vi "write includes file path.vi"(8 "error in":errorcluster, 10 "Path":path, 11 "Targets in":refnum<class "Targets.lvclass">) -> (0 "error out":errorcluster, 3 "Targets out":refnum<class "Targets.lvclass">)   [LabVIEW 2013, in "PL Framework Configuration Tool.lvlib" / "Targets.lvclass"]
uses:
  Targets.lvclass
  <vilib>/NI/Configuration Framework/serializable configuration/NISE_CEF_serializable configuration.lvclass
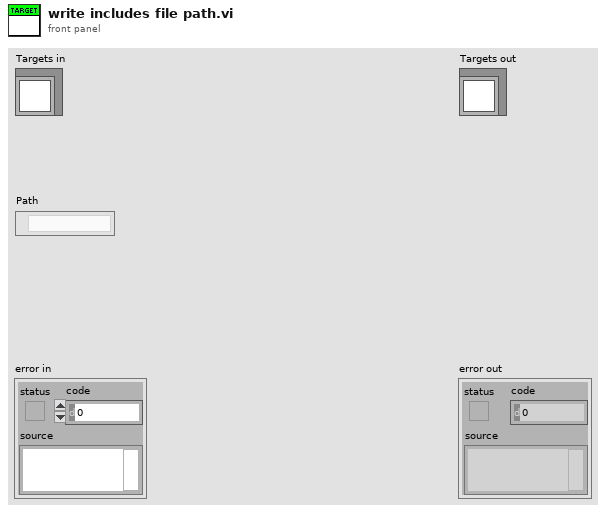
[diagram p1: front panel]
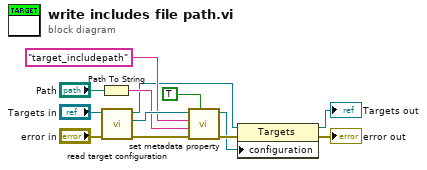
[diagram p0: block diagram]
diagram:
  n1 = Path To String(path="Path") -> (string=w6:string)
  n2 = call "read target configuration.vi"("error in"="error in", "Targets in"="Targets in") -> ("error out"=w11:errorcluster, "Target Configuration"=w9:refnum<class "PL_Target Configuration.lvclass">, "Targets out"=w3:refnum<class "Targets.lvclass">)  [unwired: 7 in]
  n3 = call <vilib>:"set metadata property.vi"("overwrite?"=TRUE, "error in"=w11, "value"=w6, "key"="target_includepath", "configuration in"=w9) -> ("error out"=w10:errorcluster, "configuration out"=w1:refnum<class "PL_Target Configuration.lvclass">)  [unwired: 5 in]
  n4 = property class="Targets"(reference=w3, error in=w10, "configuration"=w1) -> (reference out=→"Targets out":refnum<class "Targets.lvclass">, error out=→"error out":errorcluster)
